vi "ListConsoleErrors.vi"() -> (2 "Array":string[][](array[string]), 3 "Total Console Errors":i32)   [LabVIEW 2012]
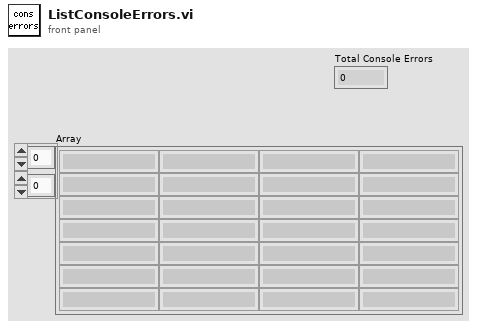
[diagram p1: front panel]
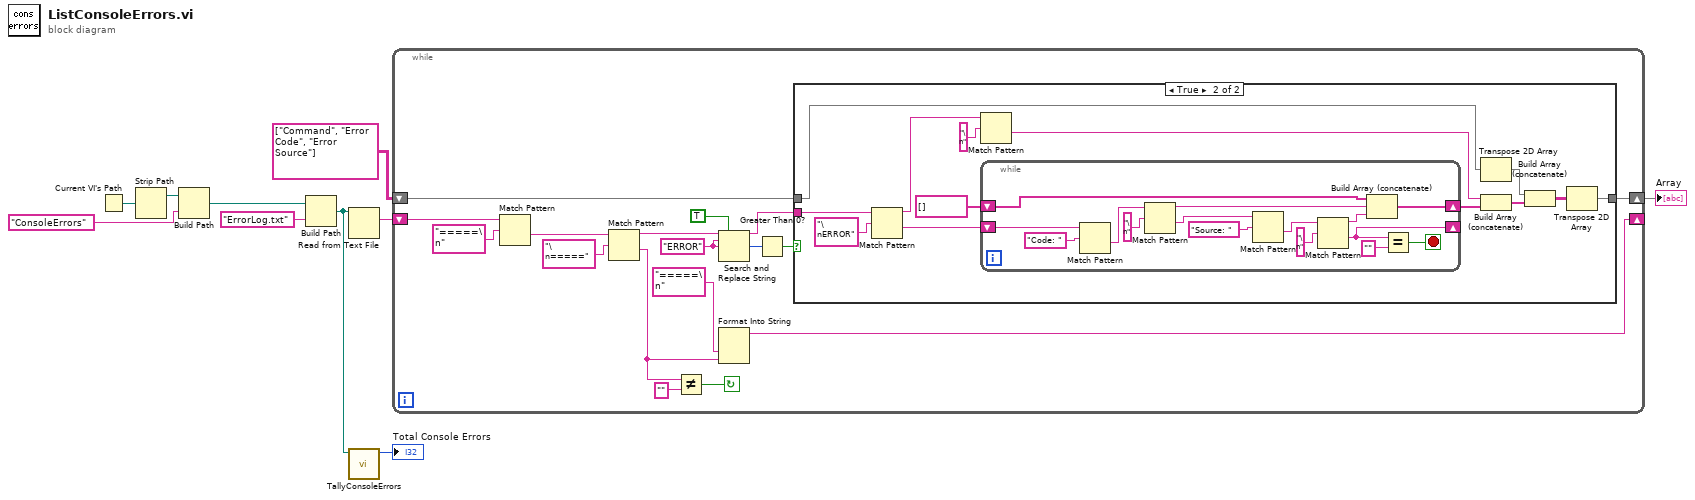
[diagram p0: block diagram]
diagram:
  n1 = Current VI's Path() -> (path=w7:path)
  n2 = Strip Path(path=w7) -> (stripped path=w6:path)  [unwired: 1 out]
  n3 = Build Path(base path=w6, name or relative path="ConsoleErrors") -> (appended path=w4:path)
  n4 = Build Path(base path=w4, name or relative path="ErrorLog.txt") -> (appended path=w2:path)
  n5 = Read from Text File(file (use dialog)=w2) -> (text=w10:string)  [unwired: 3 in, 3 out]
  n6 = call <userlib>:"TallyConsoleErrors.vi"("error log"=w2) -> ("number of errors"=→"Total Console Errors":i32)  [unwired: 10 in]
  n7 = while {
    shift-right: [w13] -> _
    shift-left: w10 -> [w24]
    shift-right: [w16] -> w8
    shift-left: string[][] [["Command"], ["Error Code"], ["Error Source"]] -> [w17]
    stop <- w15 continue-if-true
    w19 = "ERROR" ("regular expression")
    n8 = Match Pattern(string=w24, regular expression="=====\n") -> (after substring=w25:string)  [unwired: 1 in, 3 out]
    n9 = Match Pattern(string=w25, regular expression="\n=====") -> (before substring=w23:string, after substring=w11:string)  [unwired: 1 in, 2 out]
    n10 = Not Equal?(x=w11, y="") -> (x != y?=w15:bool)
    n11 = Search and Replace String(replace all?=TRUE ("replace all? (F)"), input string=w23, search string=w19, replace string=w19) -> (result string=w18:string, number of replacements=w21:i32)  [unwired: 4 in, 2 out]
    n12 = Format Into String("=====\n" ("regular expression"), w11) -> (resulting string=w13:string)  [unwired: 3 in, 1 out]
    n13 = Greater Than 0?(x=w21) -> (x > 0?=w20:bool)
    n14 = case shown="True" w20 {
      tunnel: w18 -> [_ w41]
      tunnel: w17 -> [w28 w38]
      tunnel: [w28 w32] -> w16
      frame False {
      }
      frame True {
        n15 = Match Pattern(string=w41, regular expression="\nERROR") -> (before substring=w37:string, after substring=w36:string)  [unwired: 1 in, 2 out]
        n16 = Match Pattern(string=w37, regular expression="\n") -> (after substring=w31:string)  [unwired: 1 in, 3 out]
        n17 = while {
          shift-right: [w45] -> w29
          shift-left: string[] [] ("appended array") -> [w46]
          shift-right: [w42] -> _
          shift-left: w36 -> [w49]
          stop <- w44 stop-if-true
          n18 = Match Pattern(string=w49, regular expression="Code: ") -> (after substring=w55:string)  [unwired: 1 in, 3 out]
          n19 = Match Pattern(string=w55, regular expression="\n") -> (before substring=w48:string, after substring=w50:string)  [unwired: 1 in, 2 out]
          n20 = Match Pattern(string=w50, regular expression="Source: ") -> (after substring=w52:string)  [unwired: 1 in, 3 out]
          n21 = Match Pattern(string=w52, regular expression="\n") -> (before substring=w47:string, after substring=w42:string)  [unwired: 1 in, 2 out]
          n22 = Build Array (concatenate)(w46, w48, w47) -> (w45:string[])
          n23 = Equal?(x=w42, y="") -> (x = y?=w44:bool)
        }
        n24 = Transpose 2D Array(2D array=w38) -> (transposed array=w35:string[][])
        n25 = Build Array (concatenate)(w31, w29) -> (w34:string[])
        n26 = Build Array (concatenate)(w35, w34) -> (w33:string[][])
        n27 = Transpose 2D Array(2D array=w33) -> (transposed array=w32:string[][])
      }
    }
  }
  "Array" <- w8
